vi "DrawBackground.vi"(8 "error in (no error)":errorcluster, 11 "Snake in":refnum<class "SnakeGame.lvclass">) -> (0 "error out":errorcluster, 3 "Snake out":refnum<class "SnakeGame.lvclass">)   [LabVIEW 2019, in "RT_Game.lvlib" / "SnakeGame.lvclass"]
uses:
  SnakeGame.lvclass
  C:/Users/FreshBob/Dropbox/VIs/myRIO_GameConsole/RT/RT_Game/Game/Game.lvclass
  Game/Coordinate.ctl
  SnakeGame.lvclass/SnakeGame.ctl
  Game/Game.lvclass
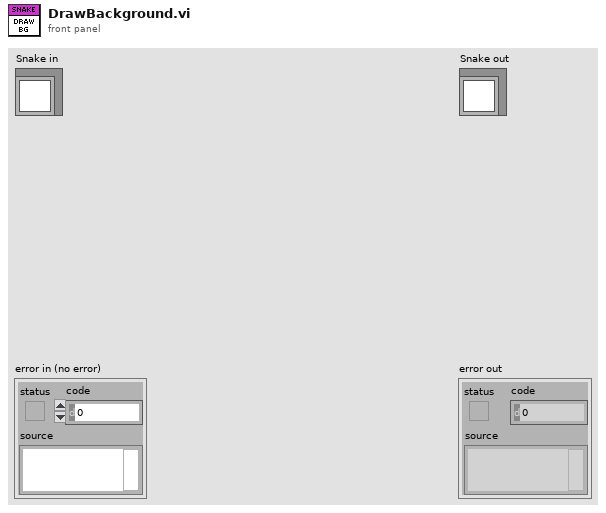
[diagram p1: front panel]
types:
  T1 = typedef "RT_Game.lvlib/Game.lvclass/Coordinate.ctl" = cluster{"x":dbl, "y":dbl}
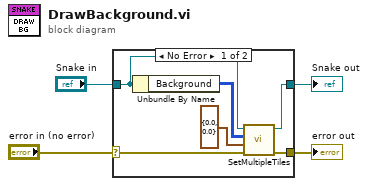
[diagram p0: block diagram]
diagram:
  n1 = case shown="No Error" "error in (no error)" {
    selector: "error in (no error)" -> [w10 w12]
    tunnel: [w7 w12] -> w3
    tunnel: [w8 w11] -> w1
    tunnel: "Snake in" -> [w5 w11]
    frame No Error {
      n2 = Unbundle By Name(w5) -> ("Background"=w9:u32[][])
      n3 = call "SetMultipleTiles.vi"("error in (no error)"=w10, "Position"=T1 {"x"=0.0, "y"=0.0}, "TileCodes"=w9, "Game in"=w5) -> ("error out"=w7:errorcluster, "Game out"=w8:refnum<class "SnakeGame.lvclass">)  [unwired: 6 in]
    }
    frame Error {
    }
  }
  "error out" <- w3
  "Snake out" <- w1
